vi "Notify.vi"(8 "error in (no error)":errorcluster, 10 "ErrorOrSuccess":refnum<class "ErrorOrSuccess.lvclass">, 11 "Register JSON in":refnum<class "Register JSON.lvclass">) -> (0 "error out":errorcluster, 3 "Register JSON out":refnum<class "Register JSON.lvclass">)   [LabVIEW 2020, in "wamplv.lvlib" / "Register JSON.lvclass"]
uses:
  Register JSON.lvclass
  Register JSON.lvclass/Register JSON.ctl
  Message loop classes/ErrorOrSuccess JSON/ErrorOrSuccess JSON.lvclass
  Message loop classes/ErrorOrSuccess/ErrorOrSuccess.lvclass
  C:/local/wamplv/Private/Message loop classes/ErrorOrSuccess/ErrorOrSuccess.lvclass
  C:/local/wamplv/Private/Message loop classes/ErrorOrSuccess JSON/ErrorOrSuccess JSON.lvclass
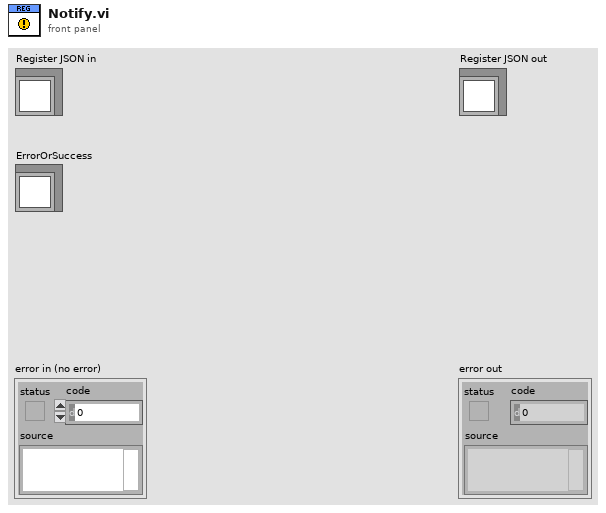
[diagram p1: front panel]
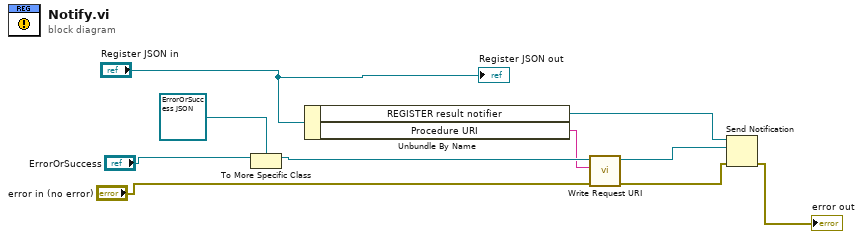
[diagram p0: block diagram]
diagram:
  n1 = To More Specific Class(target class=refnum<class "ErrorOrSuccess JSON.lvclass"> refnum ("wamplv.lvlib:ErrorOrSuccess JSON.lvclass"), reference="ErrorOrSuccess") -> (specific class reference=w6:refnum<class "ErrorOrSuccess JSON.lvclass">)  [unwired: 1 in, 1 out]
  n2 = Unbundle By Name("Register JSON in") -> ("REGISTER result notifier"=w9:refnum<notifier>, "Procedure URI"=w2:string)
  n3 = call "Write Request URI.vi"("error in (no error)"="error in (no error)", "Request URI"=w2, "ErrorOrSuccess in"=w6) -> ("error out"=w5:errorcluster, "ErrorOrSuccess out"=w1:refnum<class "ErrorOrSuccess JSON.lvclass">)  [unwired: 7 in]
  n4 = Send Notification(notification=w1, notifier=w9, error in (no error)=w5) -> (error out=→"error out":errorcluster)  [unwired: 1 out]
  "Register JSON out" <- "Register JSON in"
